vi "getData.vi"(8 "error in (no error)":errorcluster, 10 "device_name":string, 11 "ScriptEventList in":refnum<class "ScriptEventList.lvclass">) -> (0 "error out":errorcluster, 1 "singleToneData":T2(array[cluster]), 2 "data out":T3(array[cluster]), 3 "ScriptEventList out":refnum<class "ScriptEventList.lvclass">, 4 "dataType":T1(ring))   [LabVIEW 2009, in "Tools.lvlib" / "Scripting.lvlib" / "ScriptEventList.lvclass"]
uses:
  ScriptEventList.lvclass
  DatabaseHelpers/Database Objects/Channel/Channel.lvclass
  ScriptEventList.lvclass/ScriptEventList.ctl
  ScriptEvent.lvclass
  ScriptEvents/SingleTone/SingleTone.lvclass
panel:
  out "out":dbl[](array[numeric])
  out "in":dbl[](array[numeric])
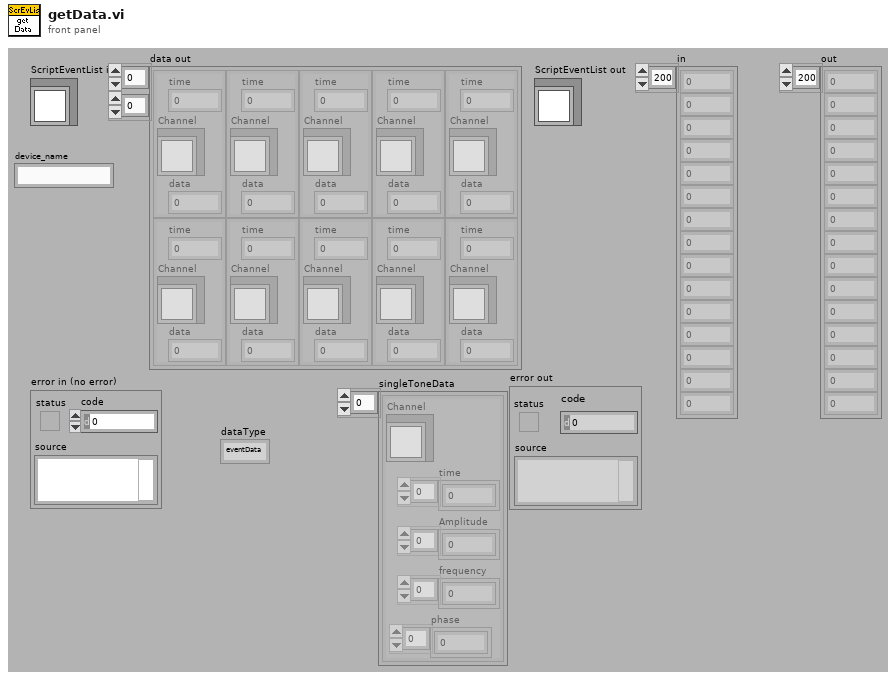
[diagram p1: front panel]
types:
  T1 = enum16{"eventData", "singleToneData", "fileData"}
  T2 = cluster{"Channel":refnum<class "Channel.lvclass">, "time":dbl[], "Amplitude":dbl[], "frequency":dbl[], "phase":dbl[]}[]
  T3 = cluster{"time":dbl, "Channel":refnum<class "Channel.lvclass">, "data":dbl}[][]
  T4 = cluster{"times":dbl[], "Channel":refnum<class "Channel.lvclass">, "data":dbl[]}
  T5 = cluster{"Tools.lvlib:DatabaseHelpers.lvlib:Channel.lvclass":refnum<class "Channel.lvclass">, "time":dbl[], "Amplitude":dbl[], "frequency":dbl[], "phase":dbl[]}[]
  T6 = cluster{dbl, "Channel":refnum<class "Channel.lvclass">, dbl}[][]
  T7 = cluster{"time":dbl, "Channel":refnum<class "Channel.lvclass">, "value":dbl}[][]
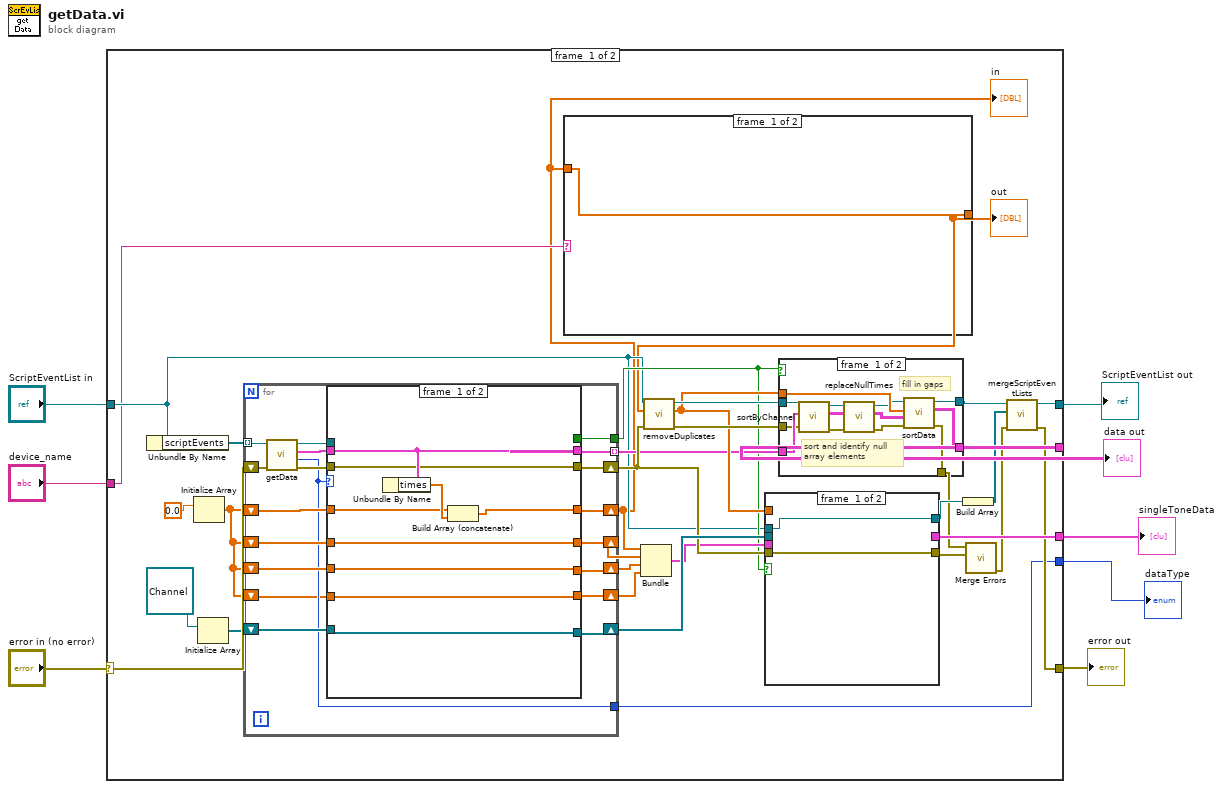
[diagram p0: block diagram]
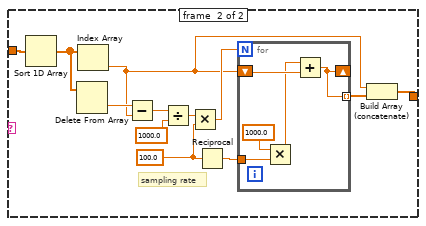
[diagram p2: hidden frame]
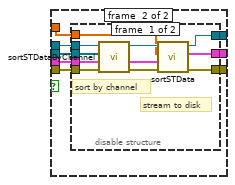
[diagram p3: hidden frame]
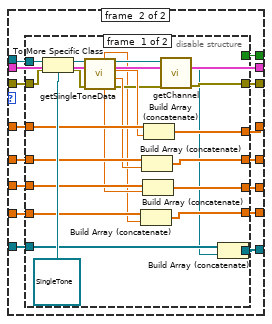
[diagram p6: hidden frame]
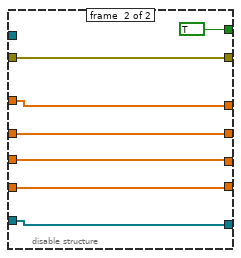
[diagram p7: hidden frame]
diagram:
  n1 = case shown="No Error" "error in (no error)" {
    selector: "error in (no error)" -> [w39 w171]
    tunnel: [w16 w171] -> w7
    tunnel: [w22 w170] -> w5
    tunnel: "ScriptEventList in" -> [w12 w170]
    tunnel: [w36 _] -> w4
    tunnel: [w25 _] -> w3
    tunnel: [w15 _] -> w2
    tunnel: "device_name" -> [w11 _]
    frame #0 {
      n2 = Unbundle By Name(w12) -> ("scriptEvents"=w40:refnum<class "ScriptEvent.lvclass">[])
      n3 = Initialize Array(0.0) -> (w14:dbl[])  [unwired: 1 in]
      n4 = Initialize Array(refnum<class "Channel.lvclass"> refnum ("Tools.lvlib:DatabaseHelpers.lvlib:Channel.lvclass")) -> (w33:refnum<class "Channel.lvclass">[])  [unwired: 1 in]
      n5 = for {
        tunnel: w40 -> [w115] mode=indexing
        shift-right: [w108] -> w30
        shift-left: w39 -> [w114]
        tunnel: [w110] -> w27 mode=indexing
        shift-right: [w112] -> w10
        shift-left: w14 -> [w113]
        shift-right: [w105] -> w32
        shift-left: w14 -> [w106]
        shift-right: [w104] -> w26
        shift-left: w14 -> [w103]
        shift-right: [w101] -> w31
        shift-left: w33 -> [w102]
        tunnel: [w100] -> w24
        tunnel: [w99] -> w15
        shift-right: [w97] -> w13
        shift-left: w14 -> [w98]
        n6 = call-dynamic "getData.vi"("error in (no error)"=w114, "ScriptEvent in"=w115) -> ("error out"=w109:errorcluster, "dataType"=w99:T1, "data"=w111:T4, "ScriptEvent out"=w107:refnum<class "ScriptEvent.lvclass">)  [unwired: 6 in]
        n7 = case shown="\"eventData\", Default" w99 {
          tunnel: w113 -> [w123 w137]
          tunnel: [w122 w138] -> w112
          tunnel: w111 -> [w121 w125]
          tunnel: [w121 w125] -> w110
          tunnel: w109 -> [w120 w136]
          tunnel: [w120 w131] -> w108
          tunnel: w107 -> [_ w139]
          tunnel: w106 -> [w119 w135]
          tunnel: [w119 w134] -> w105
          tunnel: [w118 w133] -> w104
          tunnel: w103 -> [w118 w132]
          tunnel: w102 -> [w116 w130]
          tunnel: [w116 w129] -> w101
          tunnel: [_ w128] -> w100
          tunnel: w98 -> [w117 w127]
          tunnel: [w117 w126] -> w97
          frame #0 {
            n8 = Unbundle By Name(w121) -> ("times"=w124:dbl[])
            n9 = Build Array (concatenate)(w123, w124) -> (w122:dbl[])
          }
          frame #1 {
            n10 = disable-structure shown="Enabled" {
              disable-tunnel: w139 -> [w162 _]
              disable-tunnel: [w158 w168] -> w138
              disable-tunnel: w137 -> [w157 w168]
              disable-tunnel: w136 -> [w155 w164]
              disable-tunnel: w135 -> [w154 w167]
              disable-tunnel: [w153 w167] -> w134
              disable-tunnel: [w151 w166] -> w133
              disable-tunnel: w132 -> [w150 w166]
              disable-tunnel: [w146 w164] -> w131
              disable-tunnel: w130 -> [w145 w163]
              disable-tunnel: [w144 w163] -> w129
              disable-tunnel: [_ TRUE] -> w128
              disable-tunnel: w127 -> [w143 w165]
              disable-tunnel: [w142 w165] -> w126
              frame #0 {
                n11 = To More Specific Class(target class=refnum<class "SingleTone.lvclass"> refnum ("Tools.lvlib:Scripting.lvlib:SingleTone.lvclass"), reference=w162, error in=w155) -> (specific class reference=w160:refnum<class "SingleTone.lvclass">, error out=w159:errorcluster)
                n12 = call "getSingleToneData.vi"("error in (no error)"=w159, "SingleTone in"=w160) -> ("error out"=w147:errorcluster, "amplitude"=w152:dbl, "time"=w156:dbl, "SingleTone out"=w148:refnum<class "SingleTone.lvclass">, "frequency"=w149:dbl, "phase"=w141:dbl)  [unwired: 4 in]
                n13 = Build Array (concatenate)(w143, w141) -> (w142:dbl[])
                n14 = Build Array (concatenate)(w154, w152) -> (w153:dbl[])
                n15 = Build Array (concatenate)(w150, w149) -> (w151:dbl[])
                n16 = Build Array (concatenate)(w157, w156) -> (w158:dbl[])
                n17 = call-dynamic "getChannel.vi"("error in (no error)"=w147, "ScriptEvent.lvclass in"=w148) -> ("error out"=w146:errorcluster, "Channel.lvclass"=w140:refnum<class "Channel.lvclass">)  [unwired: 7 in, 1 out]
                n18 = Build Array (concatenate)(w145, w140) -> (w144:refnum<class "Channel.lvclass">[])
              }
              frame #1 {
              }
            }
          }
        }
      }
      "in" <- w10
      n19 = case shown="\"Daq\"" w11 {
        tunnel: [w41 w43] -> w9
        tunnel: w10 -> [w41 w45]
        frame #0 {
        }
        frame #1 {
          w48 = 100.0
          # "sampling rate"
          n20 = Sort 1D Array(array=w45) -> (sorted array=w53:dbl[])
          n21 = Delete From Array(array=w53) -> (deleted portion=w52:dbl)  [unwired: 2 in, 1 out]
          n22 = Index Array(array=w53) -> (element=w42:dbl)  [unwired: 1 in]
          n23 = Subtract(x=w52, y=w42) -> (x-y=w51:dbl)
          n24 = Divide(x=w51, y=1000.0) -> (x/y=w49:dbl)
          n25 = Multiply(x=w49, y=w48) -> (x*y=w46:dbl)
          n26 = Reciprocal(x=w48) -> (1/x=w47:dbl)
          n27 = for {
            N: w46 -> [_]
            tunnel: w47 -> [w57]
            tunnel: [w54] -> w44 mode=indexing
            shift-right: [w54] -> _
            shift-left: w42 -> [w58]
            n28 = Multiply(x=1000.0, y=w57) -> (x*y=w55:dbl)
            n29 = Add(x=w55, y=w58) -> (x+y=w54:dbl)
          }
          n30 = Build Array (concatenate)(w42, w44) -> (w43:dbl[])
        }
      }
      "out" <- w9
      n31 = Bundle(w10, w32, w26, w13) -> (w29:cluster{dbl[], dbl[], dbl[], dbl[]})  [unwired: 1 in]
      n32 = call "removeDuplicates.vi"("error in (no error)"=w30, "times"=w9, "ScriptEventList in"=w12) -> ("error out"=w35:errorcluster, "times out"=w28:dbl[], "ScriptEventList out"=w37:refnum<class "ScriptEventList.lvclass">)  [unwired: 6 in]
      n33 = case shown="True" w24 {
        tunnel: w12 -> [w60 w68]
        tunnel: w31 -> [_ w67]
        tunnel: w30 -> [w59 w66]
        tunnel: w29 -> [_ w65]
        tunnel: w28 -> [_ w64]
        tunnel: [_ w63] -> w25
        tunnel: [w60 w62] -> w21
        tunnel: [w59 w61] -> w18
        frame #0 {
        }
        frame #1 {
          n34 = disable-structure shown="Enabled" {
            disable-tunnel: w68 -> [w79 w80]
            disable-tunnel: w67 -> [w78 _]
            disable-tunnel: w66 -> [w77 w81]
            disable-tunnel: w65 -> [w76 _]
            disable-tunnel: w64 -> [w73 _]
            disable-tunnel: [w71 _] -> w63
            disable-tunnel: [w70 w80] -> w62
            disable-tunnel: [w69 w81] -> w61
            frame #0 {
              # "stream to disk"
              # "sort by channel"
              n35 = call "sortSTDataByChannel.vi"("error in (no error)"=w77, "data"=w76, "channels"=w78, "ScriptEventList in"=w79) -> ("error out"=w72:errorcluster, "channelData"=w74:T5, "ScriptEventList out"=w75:refnum<class "ScriptEventList.lvclass">)  [unwired: 5 in]
              n36 = call "sortSTData.vi"("error in (no error)"=w72, "channelData"=w74, "times"=w73, "ScriptEventList in"=w75) -> ("error out"=w69:errorcluster, "sortedData"=w71:T2, "ScriptEventList out"=w70:refnum<class "ScriptEventList.lvclass">)  [unwired: 5 in]
            }
            frame #1 {
            }
          }
        }
      }
      n37 = case shown="False" w24 {
        tunnel: [w94 w96] -> w23
        tunnel: w37 -> [w93 w96]
        tunnel: w27 -> [w92 _]
        tunnel: [w91 _] -> w36
        tunnel: w35 -> [w90 w95]
        tunnel: [w89 w95] -> w19
        tunnel: w28 -> [w88 _]
        frame #0 {
          # "fill in gaps"
          # "sort and identify null\narray elements"
          n38 = call "sortByChannel.vi"("error in (no error)"=w90, "Array"=w92, "ScriptEventList in"=w93) -> ("error out"=w83:errorcluster, "data"=w87:T6, "ScriptEventList out"=w85:refnum<class "ScriptEventList.lvclass">)  [unwired: 6 in]
          n39 = call "replaceNullTimes.vi"("error in (no error)"=w83, "data in"=w87, "ScriptEventList in"=w85) -> ("error out"=w82:errorcluster, "data out"=w86:T7, "ScriptEventList out"=w84:refnum<class "ScriptEventList.lvclass">)  [unwired: 6 in]
          n40 = call "sortData.vi"("error in (no error)"=w82, "data"=w86, "times"=w88, "ScriptEventList in"=w84) -> ("error out"=w89:errorcluster, "data out"=w91:T3, "ScriptEventList out"=w94:refnum<class "ScriptEventList.lvclass">)  [unwired: 5 in]
        }
        frame #1 {
        }
      }
      n41 = Build Array(w21) -> (w20:refnum<class "ScriptEventList.lvclass">[])
      n42 = call <vilib>:"Merge Errors.vi"("error in 2 (no error)"=w18, "error in 1 (no error)"=w19) -> ("error out"=w17:errorcluster)  [unwired: 5 in]
      n43 = call "mergeScriptEventLists.vi"("error in (no error)"=w17, "Array"=w20, "ScriptEventList in"=w23) -> ("error out"=w16:errorcluster, "ScriptEventList out"=w22:refnum<class "ScriptEventList.lvclass">)  [unwired: 7 in]
    }
    frame #1 {
    }
  }
  "error out" <- w7
  "ScriptEventList out" <- w5
  "data out" <- w4
  "singleToneData" <- w3
  "dataType" <- w2
